vi "gu_string_subset.vi"(8 "error in":errorcluster, 9 "Length (rest)":i32=2147483647, 10 "Offset (0)":i32, 11 "Encoded String":T1) -> (0 "error out":errorcluster, 3 "Encoded Substring":T1)   [LabVIEW 2020, in "G-Unicode.lvlib"]
uses:
  G-Unicode.lvlib
  Types/Encoded UTF-8 String.ctl
  Memory/Copy String.vi/4d47babd-4a2d-4eb7-b91b-7e707d692665.vi
  gu_free.vi
  lib/g_unicode_32.dll
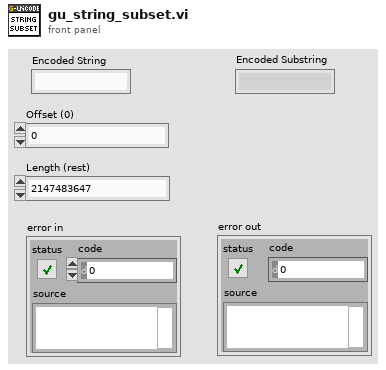
[diagram p1: front panel]
types:
  T1 = typedef "G-Unicode.lvlib/Encoded UTF-8 String.ctl" = string
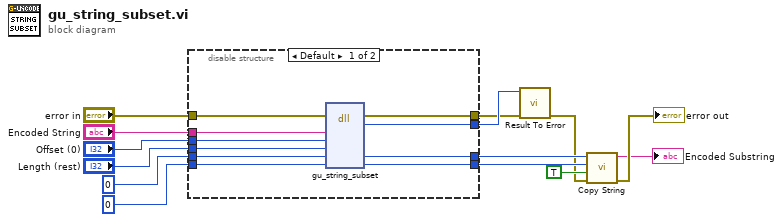
[diagram p0: block diagram]
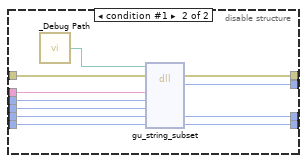
[diagram p2: hidden frame]
diagram:
  n1 = disable-structure shown="Default" {
    disable-tunnel: "Encoded String" -> [w23 w34]
    disable-tunnel: "error in" -> [w24 w35]
    disable-tunnel: [w18 w29] -> w2
    disable-tunnel: "Offset (0)" -> [w22 w33]
    disable-tunnel: "Length (rest)" -> [w21 w32]
    disable-tunnel: 0 -> [w20 w31]
    disable-tunnel: i64 0 ("substring") -> [w19 w30]
    disable-tunnel: [w17 w28] -> w6
    disable-tunnel: [w16 w27] -> w5
    disable-tunnel: [w15 w25] -> w3
    frame condition #0 (active) {
      n2 = dll-call lib="C:/github/dataflowg/g-unicode/src/LabVIEW/G-Unicode/lib/g_unicode_*.*" fn="gu_string_subset"(error in=w24, "string"=w23, "offset"=w22, "length"=w21, "substring"=w19, "substring_size"=w20) -> (error out=w18:errorcluster, "result"=w15:i32, "substring"=w17:i64, "substring_size"=w16:i32)  [unwired: 5 in, 1 out]
    }
    frame condition #1 {
      n3 = call "_Debug Path.vi"() -> ("Debug Path"=w26:path)
      n4 = dll-call lib="?" fn="gu_string_subset"(path in=w26, error in=w35, "string"=w34, "offset"=w33, "length"=w32, "substring"=w30, "substring_size"=w31) -> (error out=w29:errorcluster, "result"=w25:i32, "substring"=w28:i64, "substring_size"=w27:i32)  [unwired: 4 in, 1 out]
    }
  }
  n5 = call "Result To Error.vi"("error in (no error)"=w2, "Result Code"=w3) -> ("error out"=w1:errorcluster)  [unwired: 9 in]
  n6 = call "Copy String.vi"("error in"=w1, "free (F)"=TRUE, "size"=w5, "pointer"=w6) -> ("error out"=→"error out":errorcluster, "string"=→"Encoded Substring":string)  [unwired: 6 in]
